vi "Set id.vi"(10 "id":i32, 11 "Transfer in":refnum<class "Transfer.lvclass">) -> (3 "Transfer out":refnum<class "Transfer.lvclass">)   [LabVIEW 2017, in "DSF Core.lvlib" / "Transfer.lvclass"]
uses:
  Transfer.lvclass
  Transfer.lvclass/Transfer.ctl
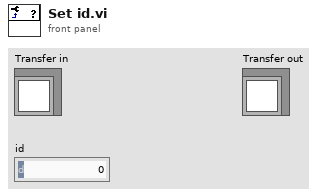
[diagram p1: front panel]
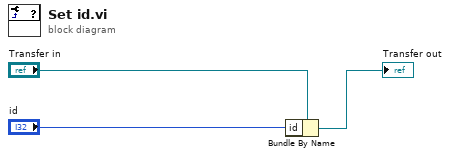
[diagram p0: block diagram]
diagram:
  n1 = Bundle By Name(cluster="Transfer in", "id"="id") -> (→"Transfer out":refnum<class "Transfer.lvclass">)
